vi "Spectrum Noise Subtraction v10.5.0.vi"(2 "Spectrum Noise":i64 caption="Noise Level", 3 "Spectrum-Array In":dbl[][](array[numeric])) -> (0 "Spectrum-Array Out":dbl[][](array[numeric]), 1 "Spectrum-Cluster":T1(array[cluster]))   [LabVIEW 2010]
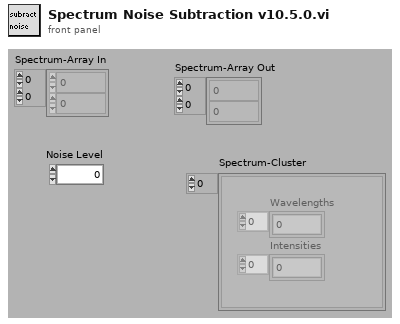
[diagram p1: front panel]
types:
  T1 = cluster{"Intensities":dbl[], "Wavelengths":dbl[]}[]
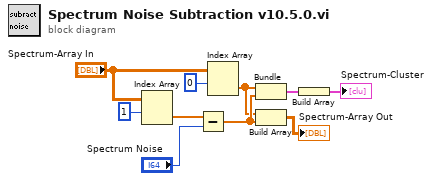
[diagram p0: block diagram]
diagram:
  n1 = Index Array(array="Spectrum-Array In", index (row)=1 ("disabled index (col)")) -> (element=w6:dbl[])  [unwired: 1 in]
  n2 = Subtract(x=w6, y="Spectrum Noise") -> (x-y=w4:dbl[])
  n3 = Index Array(array="Spectrum-Array In", index (row)=0 ("disabled index (col)")) -> (element=w3:dbl[])  [unwired: 1 in]
  n4 = Bundle("Spectrum-Array In"=w3, w4) -> (w9:cluster{"Spectrum-Array In":dbl[], dbl[]})  [unwired: 1 in]
  n5 = Build Array(w3, w4) -> (→"Spectrum-Array Out":dbl[][])
  n6 = Build Array(w9) -> (→"Spectrum-Cluster":cluster{"Spectrum-Array In":dbl[], dbl[]}[])
